vi "Gauge_Converter_TD.vi"(11 "string":string) -> (3 "TD Medio":string)   [LabVIEW 2014]
uses:
  <vilib>/ptbypt/NI_PtbyPt.lvlib
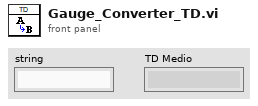
[diagram p1: front panel]
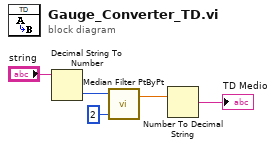
[diagram p0: block diagram]
diagram:
  n1 = Decimal String To Number(string="string") -> (number=w3:i32)  [unwired: 2 in, 1 out]
  n2 = call <vilib>:"Median Filter PtByPt.vi"("rank"=2, "x"=w3) -> ("Filtered x"=w2:dbl)  [unwired: 2 in, 1 out]
  n3 = Number To Decimal String(number=w2) -> (decimal integer string=→"TD Medio":string)  [unwired: 1 in]
